vi "Receive Message.vi"(6 "priority":i32, 10 "Instrument Handler in":refnum<class "Instrument Handler.lvclass">, 11 "Message in":refnum<class "Message.lvclass">) -> (0 "error out":errorcluster, 2 "Actor out":refnum<class "Actor.lvclass">)   [LabVIEW 2020, in "Instrument Handler.lvlib" / "Instrument Handler.lvclass"]
doc: "This implementation forwards Instrument Msgs to the other instrument processes where they are executed."
uses:
  Instrument Handler.lvclass
  PPL/HDH.Actor Framework.Core.Actor.lvlibp/1abvi3w/vi.lib/ActorFramework/Message/Message.lvclass
  PPL/HDH.Actor Framework.Core.Actor.lvlibp/1abvi3w/vi.lib/ActorFramework/Actor/Actor.lvclass
  C:/Current projects/WS/PPL/HDH.Actor Framework.Core.Actor.lvlibp/1abvi3w/vi.lib/ActorFramework/Actor/Actor.lvclass
  Messages/Instrument Msg/Instrument Msg.lvclass
  Messages/Multi Instrument Msg/Multi Instrument Msg.lvclass
  C:/Current projects/WS/Framework/Framework/Actors/Instrument Handler/Messages/Instrument Msg/Instrument Msg.lvclass
  Instrument Handler.lvclass/Instrument Handler.ctl
  Messages/Multi Instrument Msg/Multi Instrument Msg.lvclass/Multi Instrument Msg.ctl
  Messages/Multi Instrument Wrapper Msg/Multi Instrument Wrapper Msg.lvclass/Multi Instrument Wrapper Msg.ctl
  Messages/Multi Instrument Wrapper Msg/Multi Instrument Wrapper Msg.lvclass
  PPL/HDH.Data.Generic.lvlibp
  PPL/HDH.Actor Framework.Core.Actor.lvlibp/1abvi3w/vi.lib/ActorFramework/Message Enqueuer/Message Enqueuer.lvclass
  PPL/HDH.Actor Framework.Core.Instrument Driver.lvlibp/Instrument Driver/Instrument Driver.lvclass
  C:/Current projects/WS/PPL/HDH.Actor Framework.Core.Actor.lvlibp/1abvi3w/vi.lib/ActorFramework/Message/Message.lvclass
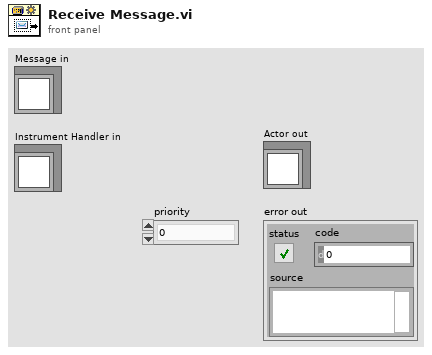
[diagram p1: front panel]
types:
  T1 = typedef "Instrument Handler.lvlib/Ctl_InstrumentSynchronicationCluster.ctl" = cluster{"Launched?":bool, "Driver Path":path, "Alias":string, "Connection Type":T2, "Pre Initialization Data":variant, "Enqueue Sync":refnum<class "Notifier.lvclass">, "Enqueue Lock":T3, "Owner Enqueuer":refnum<class "Message Enqueuer.lvclass">, "Owner":refnum<class "Sequencer Core.lvclass">, "Instrument ID":u32}
  T2 = typedef "HDH.Actor Framework.Core.Instrument Driver.lvlibp/Instrument Driver.lvclass/Ctl_ConnectionType.ctl" = enum16{"BuiltIn/System", "PXI/PCI", "USB", "GPIB", "VXI", "Serial", "TCP/IP", "cRIO", "SCXI", "cDAQ", "SwitchBlock", "SCC", "FireWire", "Accessory", "CAN", "SwitchBlock Device"}
  T3 = typedef "Semaphore RefNum" = refnum<k1>
  T4 = typedef "Instrument Handler.lvlib/Ctl_AquirerRefnum.ctl" = refnum<vi>
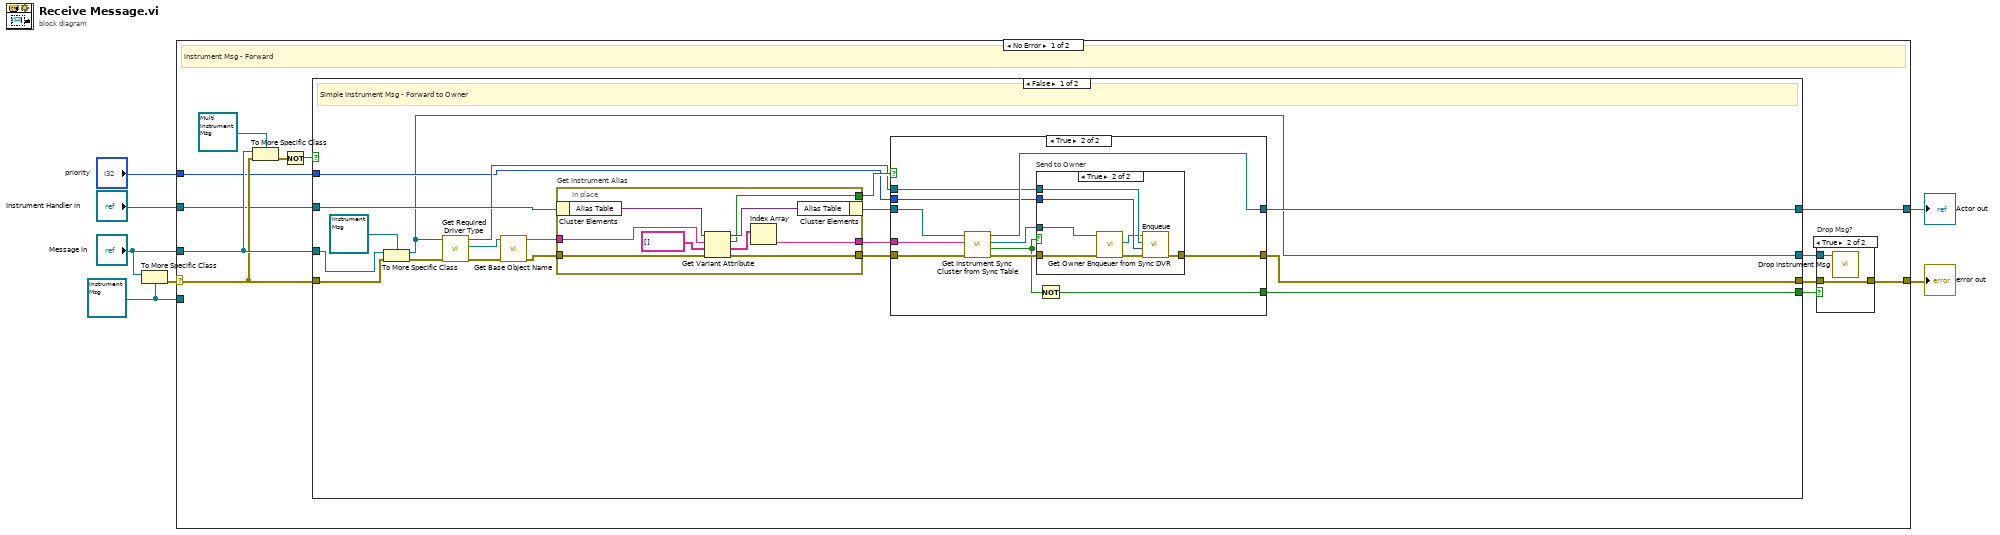
[diagram p0: block diagram]
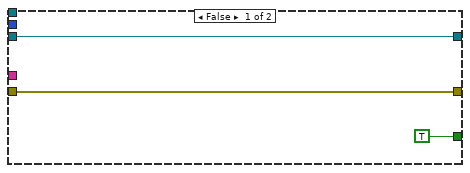
[diagram p3: hidden frame]
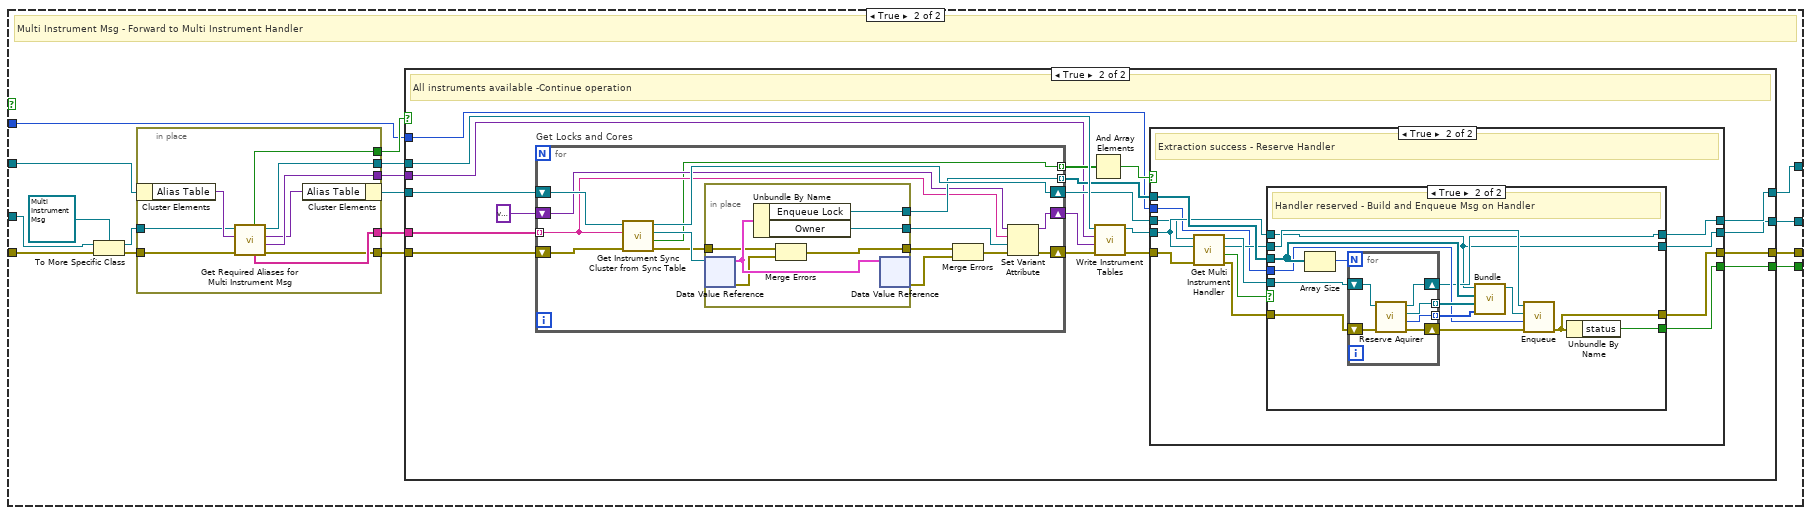
[diagram p5: hidden frame]
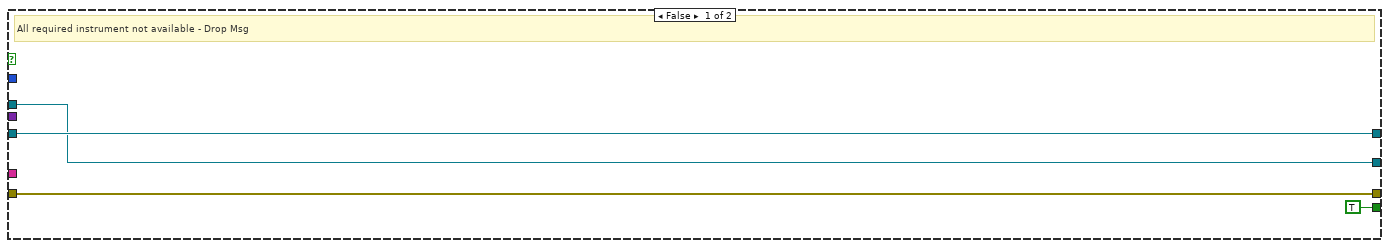
[diagram p6: hidden frame]
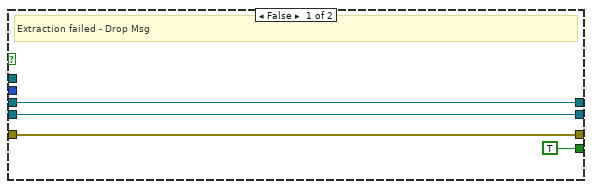
[diagram p7: hidden frame]
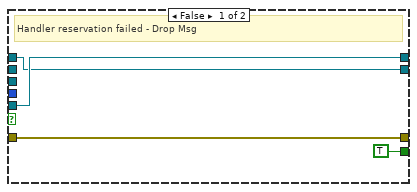
[diagram p8: hidden frame]
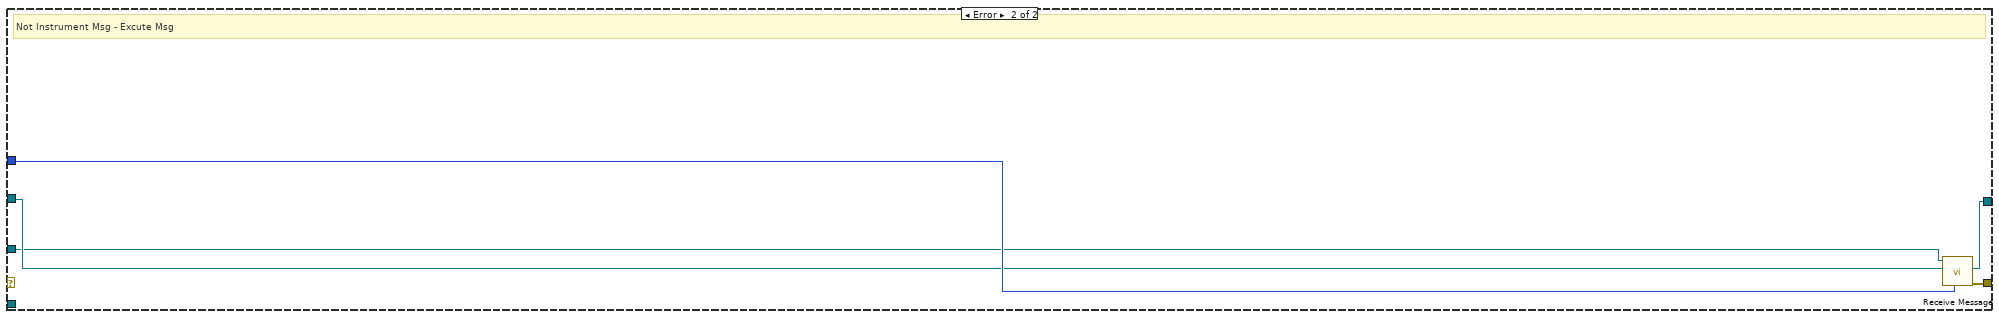
[diagram p9: hidden frame]
diagram:
  w1 = refnum<class "Instrument Msg.lvclass"> refnum ("Instrument Handler.lvlib:Instrument Msg.lvclass")
  n1 = To More Specific Class(target class=w1, reference="Message in") -> (error out=w2:errorcluster)  [unwired: 1 in, 1 out]
  n2 = case shown="No Error" w2 {
    selector: w2 -> [w15 _]
    tunnel: [w8 w188] -> w7
    tunnel: [w13 w187] -> w6
    tunnel: "priority" -> [w12 w186]
    tunnel: "Instrument Handler in" -> [w14 w185]
    tunnel: "Message in" -> [w16 w184]
    tunnel: w1 -> [_ _]
    frame No Error {
      # "Instrument Msg - Forward"
      n3 = To More Specific Class(target class=refnum<class "Multi Instrument Msg.lvclass"> refnum ("Instrument Handler.lvlib:Multi Instrument Msg.lvclass"), reference=w16, error in=w15) -> (error out=w18:errorcluster)  [unwired: 1 out]
      n4 = Not(x=w18) -> (.not. x?=w17:bool)
      n5 = case shown="False" w17 {
        tunnel: w16 -> [w41 w88]
        tunnel: w15 -> [w39 w87]
        tunnel: w14 -> [w35 w77]
        tunnel: [w30 w84] -> w13
        tunnel: [w25 w80] -> w9
        tunnel: w12 -> [w26 w78]
        tunnel: [w24 w85] -> w11
        tunnel: [w23 w83] -> w10
        frame False {
          # "Simple Instrument Msg - Forward to Owner"
          n6 = To More Specific Class(target class=refnum<class "Instrument Msg.lvclass"> refnum ("Instrument Handler.lvlib:Instrument Msg.lvclass"), reference=w41, error in=w39) -> (specific class reference=w23:refnum<class "Instrument Msg.lvclass">, error out=w38:errorcluster)
          n7 = call-dynamic "Get Required Driver Type.vi"("error in (no error)"=w38, "Instrument Msg in"=w23) -> ("error out"=w36:errorcluster, "Required Driver Type"=w37:refnum<class "Instrument Driver.lvclass">, "Instrument Msg out"=w27:refnum<class "Instrument Msg.lvclass">)  [unwired: 7 in]
          n8 = call "Get Base Object Name.vi"("error in (no error)"=w36, "Object in"=w37) -> ("error out"=w33:errorcluster, "Base class name"=w34:string)  [unwired: 8 in]
          n9 = in-place "Get instrument Alias" {
            in-place-border: w34 -> [w71]
            in-place-border: w33 -> [w69]
            in-place-border: [w67] -> w32
            in-place-border: [w66] -> w29
            in-place-border: [w64] -> w28
            n10 = in-place-cluster #1(w35) -> ("Alias Table"=w72:variant)
            n11 = Get Variant Attribute(Variant=w72, name=w71, default value (empty Variant)=string[] [] ("Base class name"), error in=w69) -> (duplicate Variant=w68:variant, found=w67:bool, value=w65:string[], error out=w66:errorcluster)
            n12 = Index Array(array=w65) -> (element=w64:string)  [unwired: 1 in]
            n13 = in-place-cluster #1("Alias Table"=w68) -> (w31:refnum<class "Instrument Handler.lvclass">)
          }
          n14 = case shown="True" w32 {
            tunnel: w31 -> [w44 w55]
            tunnel: [w44 w52] -> w30
            tunnel: [w43 w49] -> w25
            tunnel: w29 -> [w43 w53]
            tunnel: w28 -> [_ w54]
            tunnel: w27 -> [_ w51]
            tunnel: w26 -> [_ w50]
            tunnel: [TRUE ("status") w45] -> w24
            frame False {
            }
            frame True {
              n15 = call "Get Instrument Sync Cluster from Sync Table.vi"("error in (no error)"=w53, "Instrument Alias"=w54, "Instrument Handler in"=w55) -> ("error out"=w47:errorcluster, "Success?"=w46:bool, "data value reference"=w48:refnum<data-value>, "Instrument Handler out"=w52:refnum<class "Instrument Handler.lvclass">)  [unwired: 5 in]
              n16 = case "Send to Owner" shown="True" w46 {
                tunnel: w51 -> [_ w63]
                tunnel: w50 -> [_ w62]
                tunnel: [w56 w61] -> w49
                tunnel: w48 -> [_ w60]
                tunnel: w47 -> [w56 w58]
                frame False {
                }
                frame True {
                  n17 = call "Get Owner Enqueuer from Sync DVR.vi"("error in (no error)"=w58, "Data Value Reference in"=w60) -> ("error out"=w57:errorcluster, "Owner Enqueuer"=w59:refnum<class "Message Enqueuer.lvclass">)  [unwired: 7 in, 1 out]
                  n18 = call "Enqueue.vi"("error in (no error)"=w57, "Message Priority (Normal)"=w62, "Message"=w63, "Message Enqueuer in"=w59) -> ("error out"=w61:errorcluster)  [unwired: 6 in, 1 out]
                }
              }
              n19 = Not(x=w46) -> (.not. x?=w45:bool)
            }
          }
        }
        frame True {
          # "Multi Instrument Msg - Forward to Multi Instrument Handler"
          n20 = To More Specific Class(target class=refnum<class "Multi Instrument Msg.lvclass"> refnum ("Instrument Handler.lvlib:Multi Instrument Msg.lvclass"), reference=w88, error in=w87) -> (specific class reference=w74:refnum<class "Multi Instrument Msg.lvclass">, error out=w75:errorcluster)
          n21 = in-place {
            in-place-border: w75 -> [w92]
            in-place-border: [w98] -> w86
            in-place-border: [w97] -> w82
            in-place-border: [w96] -> w81
            in-place-border: [w91] -> w79
            in-place-border: w74 -> [w94]
            in-place-border: [w93] -> w73
            n22 = in-place-cluster #2(w77) -> ("Alias Table"=w95:variant)
            n23 = call "Get Required Aliases for Multi Instrument Msg.vi"("error in (no error)"=w92, "Alias Table in"=w95, "Multi Instrument Msg in"=w94) -> ("error out"=w96:errorcluster, "Alias Sub Table"=w91:variant, "Alias Table out"=w90:variant, "Multi Instrument Msg out"=w93:refnum<class "Multi Instrument Msg.lvclass">, "Alias Array"=w97:string[], "All Instruments Present?"=w98:bool)  [unwired: 3 in]
            n24 = in-place-cluster #2("Alias Table"=w90) -> (w76:refnum<class "Instrument Handler.lvclass">)
          }
          n25 = case shown="True" w86 {
            tunnel: [TRUE w112] -> w85
            tunnel: [w101 w110] -> w84
            tunnel: w76 -> [w101 w121]
            tunnel: [w100 w107] -> w83
            tunnel: w73 -> [w100 w117]
            tunnel: w82 -> [_ w120]
            tunnel: w81 -> [w99 w119]
            tunnel: [w99 w109] -> w80
            tunnel: w79 -> [_ w103]
            tunnel: w78 -> [_ w104]
            frame False {
              # "All required instrument not available - Drop Msg"
            }
            frame True {
              # "All instruments available -Continue operation"
              n26 = for "Get Locks and Cores" {
                shift-right: [w176] -> w111
                shift-left: w121 -> [w177]
                tunnel: w120 -> [w171] mode=indexing
                shift-right: [w165] -> w115
                shift-left: w119 -> [w175]
                shift-right: [w164] -> w116
                shift-left: variant -> [w172]
                tunnel: [w173] -> w105 mode=indexing
                tunnel: [w163] -> w114 mode=indexing
                n27 = call "Get Instrument Sync Cluster from Sync Table.vi"("error in (no error)"=w175, "Instrument Alias"=w171, "Instrument Handler in"=w177) -> ("error out"=w169:errorcluster, "Success?"=w163:bool, "data value reference"=w174:refnum<data-value>, "Instrument Handler out"=w176:refnum<class "Instrument Handler.lvclass">)  [unwired: 5 in]
                n28 = in-place {
                  in-place-border: [w182] -> w173
                  in-place-border: [w181] -> w170
                  in-place-border: w169 -> [w180]
                  in-place-border: [w178] -> w168
                  n29 = in-place-dvr #3(w174) -> (w183:T1, w179:errorcluster)
                  n30 = Unbundle By Name(w183) -> ("Enqueue Lock"=w182:T3, "Owner"=w181:refnum<class "Sequencer Core.lvclass">)
                  n31 = Merge Errors(w180, w179) -> (w178:errorcluster)
                  n32 = in-place-dvr #3(w183) -> (w167:errorcluster)  [unwired: 1 out]
                }
                n33 = Merge Errors(w168, w167) -> (w166:errorcluster)
                n34 = Set Variant Attribute(Variant=w172, name=w171, value=w170, error in=w166) -> (Variant out=w164:variant, error out=w165:errorcluster)  [unwired: 1 out]
              }
              n35 = And Array Elements(Boolean array=w114) -> (logical AND=w113:bool)
              n36 = call "Write Instrument Tables.vi"("error in (no error)"=w115, "Core Table"=w116, "Alias Table"=w103, "Multi Instrument Msg in"=w117) -> ("error out"=w108:errorcluster, "Multi Instrument Msg out"=w106:refnum<class "Multi Instrument Msg.lvclass">)  [unwired: 6 in]
              n37 = case shown="True" w113 {
                tunnel: [TRUE w127] -> w112
                tunnel: [w124 w128] -> w110
                tunnel: w111 -> [w124 w136]
                tunnel: [w123 w129] -> w109
                tunnel: w108 -> [w123 w134]
                tunnel: [w122 w126] -> w107
                tunnel: w106 -> [w122 w137]
                tunnel: w105 -> [_ w138]
                tunnel: w104 -> [_ w130]
                frame False {
                  # "Extraction failed - Drop Msg"
                }
                frame True {
                  # "Extraction success - Reserve Handler"
                  n38 = call "Get Multi Instrument Handler.vi"("error in (no error)"=w134, "Msg"=w137, "Instrument Handler in"=w136) -> ("error out"=w133:errorcluster, "Success?"=w132:bool, "Enqueuer"=w131:refnum<class "Message Enqueuer.lvclass">, "Instrument Handler out"=w135:refnum<class "Instrument Handler.lvclass">)  [unwired: 5 in]
                  n39 = case shown="True" w132 {
                    tunnel: w138 -> [_ w155]
                    tunnel: w137 -> [w139 w143]
                    tunnel: w135 -> [w140 w152]
                    tunnel: w133 -> [w141 w151]
                    tunnel: w131 -> [_ w149]
                    tunnel: w130 -> [_ w148]
                    tunnel: [w141 w145] -> w129
                    tunnel: [w140 w146] -> w128
                    tunnel: [TRUE w144] -> w127
                    tunnel: [w139 w143] -> w126
                    frame False {
                      # "Handler reservation failed - Drop Msg"
                    }
                    frame True {
                      # "Handler reserved - Build and Enqueue Msg on Handler"
                      n40 = Array Size(array=w155) -> (size(s)=w156:i32)
                      n41 = for {
                        N: w156 -> [_]
                        shift-right: [w161] -> w146
                        shift-left: w152 -> [w162]
                        shift-right: [w159] -> w147
                        shift-left: w151 -> [w160]
                        tunnel: [w158] -> w153 mode=indexing
                        tunnel: [w157] -> w154 mode=indexing
                        n42 = call "Reserve Aquirer.vi"("error in (no error)"=w160, "Instrument Handler in"=w162) -> ("error out"=w159:errorcluster, "Aquirer Index"=w157:i32, "Aquirer"=w158:T4, "Instrument Handler out"=w161:refnum<class "Instrument Handler.lvclass">)  [unwired: 6 in]
                      }
                      n43 = call "Bundle.vi"("Aquirer Indices"=w154, "Aquirer"=w153, "Enqueue Locks"=w155, "Msg"=w143) -> ("Multi Instrument Wrapper Msg out"=w150:refnum<class "Multi Instrument Wrapper Msg.lvclass">)  [unwired: 7 in]
                      n44 = call "Enqueue.vi"("error in (no error)"=w147, "Message Priority (Normal)"=w148, "Message"=w150, "Message Enqueuer in"=w149) -> ("error out"=w145:errorcluster)  [unwired: 6 in, 1 out]
                      n45 = Unbundle By Name(w145) -> ("status"=w144:bool)
                    }
                  }
                }
              }
            }
          }
        }
      }
      n46 = case "Drop Msg?" shown="True" w11 {
        tunnel: w10 -> [_ w22]
        tunnel: w9 -> [w20 w21]
        tunnel: [w20 w21] -> w8
        frame False {
        }
        frame True {
          n47 = call "Drop Instrument Msg.vi"("Instrument Msg in"=w22) -> ()  [unwired: 11 in]
        }
      }
    }
    frame Error {
      # "Not Instrument Msg - Excute Msg"
      n48 = call-parent "Receive Message.vi"("priority"=w186, "Actor in"=w185, "Message in"=w184) -> ("error out"=w188:errorcluster, "Actor out"=w187:refnum<class "Actor.lvclass">)  [unwired: 7 in]
    }
  }
  "error out" <- w7
  "Actor out" <- w6
